vi "TimeStamp.vi"(8 "Root Path":path, 11 "Build Name":string="NONE") -> (0 "filename string":string, 1 "Directory Path":path, 3 "File Path":path)   [LabVIEW 2017]
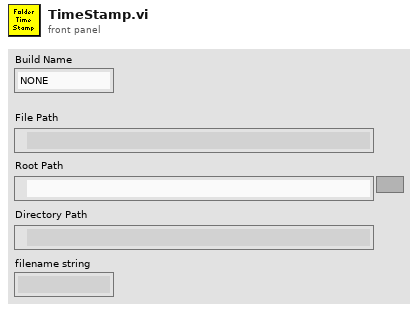
[diagram p1: front panel]
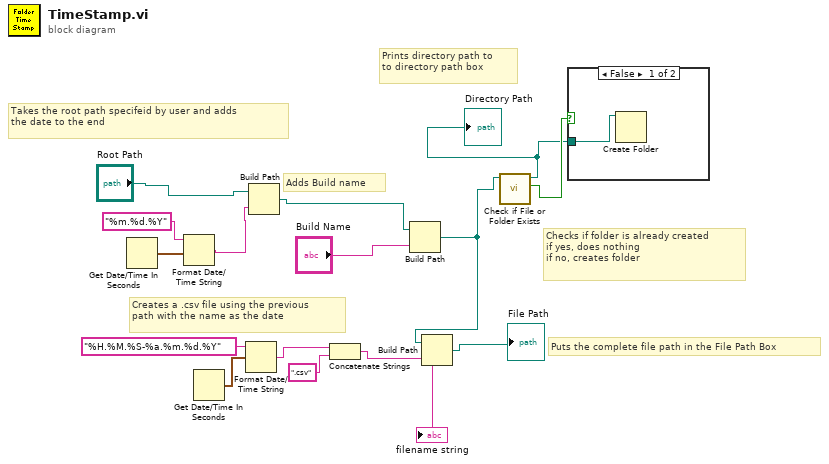
[diagram p0: block diagram]
diagram:
  # "Prints directory path to\nto directory path box"
  # "Checks if folder is already created\nif yes, does nothing\nif no, creates folder"
  # "Puts the complete file path in the File Path Box"
  # "Creates a .csv file using the previous\npath with the name as the date"
  # "Adds Build name"
  # "Takes the root path specifeid by user and adds\nthe date to the end"
  n1 = Get Date/Time In Seconds() -> (seconds since 1Jan1904=w5:timestamp)
  n2 = Format Date/Time String(time format string (%c)="%m.%d.%Y", seconds (now)=w5) -> (date/time string=w3:string)  [unwired: 1 in]
  n3 = Get Date/Time In Seconds() -> (seconds since 1Jan1904=w14:timestamp)
  n4 = Format Date/Time String(time format string (%c)="%H.%M.%S-%a.%m.%d.%Y", seconds (now)=w14) -> (date/time string=w13:string)  [unwired: 1 in]
  n5 = Build Path(base path="Root Path", name or relative path=w3) -> (appended path=w1:path)
  n6 = Concatenate Strings(w13, ".csv" ("string")) -> (w11:string)
  "filename string" <- w11
  n7 = Build Path(base path=w1, name or relative path="Build Name") -> (appended path=w8:path)
  n8 = Build Path(base path=w8, name or relative path=w11) -> (appended path=→"File Path":path)
  n9 = call <vilib>:"Check if File or Folder Exists.vi"("path"=w8) -> ("file or folder exists?"=w9:bool, "dup path"=w6:path)  [unwired: 8 in, 1 out]
  "Directory Path" <- w6
  n10 = case shown="False" w9 {
    tunnel: w6 -> [w16 _]
    frame False {
      n11 = Create Folder(path (use dialog)=w16) -> ()  [unwired: 2 in, 3 out]
    }
    frame True {
    }
  }
